vi "Packet Transmit Loop.vi"   [LabVIEW 2015]
uses:
  Packet Transmitter Action.ctl
types:
  T1 = typedef "Packet Transmitter Action.ctl" = enum16{"Initialize", "Enqueue for Send", "Retrieve for Send"}
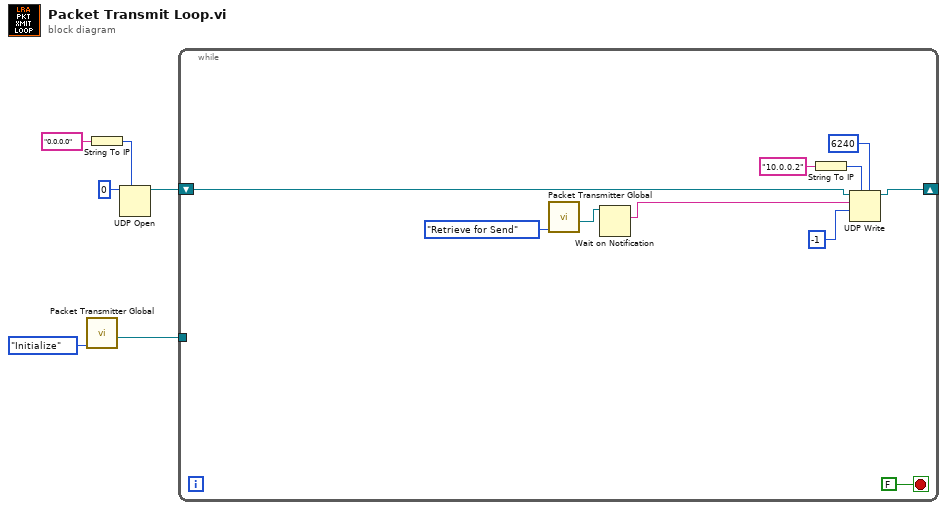
[diagram p0: block diagram]
diagram:
  n1 = call "Packet Transmitter Global.vi"("Action"=Packet_Transmitter_Action."Initialize") -> ("notifier out"=w1:refnum<notifier>)  [unwired: 10 in]
  n2 = String To IP(1:"0.0.0.0" ("name")) -> (0:w6:u32)
  n3 = UDP Open(7:w6, 11:u16 0 ("port")) -> (port=w4:refnum<k16>)  [unwired: 3 in, 2 out]
  n4 = while {
    shift-right: [w14] -> _
    shift-left: w4 -> [w15]
    tunnel: w1 -> [_]
    stop <- FALSE stop-if-true
    n5 = call "Packet Transmitter Global.vi"("Action"=Packet_Transmitter_Action."Retrieve for Send") -> ("notifier out"=w8:refnum<notifier>)  [unwired: 10 in]
    n6 = Wait on Notification(notifier=w8) -> (notification=w7:string)  [unwired: 3 in, 3 out]
    n7 = String To IP(1:"10.0.0.2" ("name")) -> (0:w10:u32)
    n8 = UDP Write(address=w10, port or service name=u16 6240, connection ID=w15, data in=w7, 9:-1 ("timeout ms (25000)")) -> (3:w14:refnum<k16>)  [unwired: 1 in, 1 out]
  }
